vi "zad3.vi"() -> ()   [LabVIEW 2017]
panel:
  in  "Tryb awaryjny":bool
  in  "stop":bool
  out "Lampa Uliczna":cluster{"1":bool, "2":bool, "3":bool}
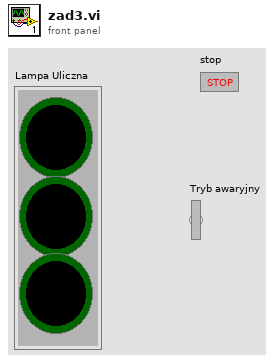
[diagram p1: front panel]
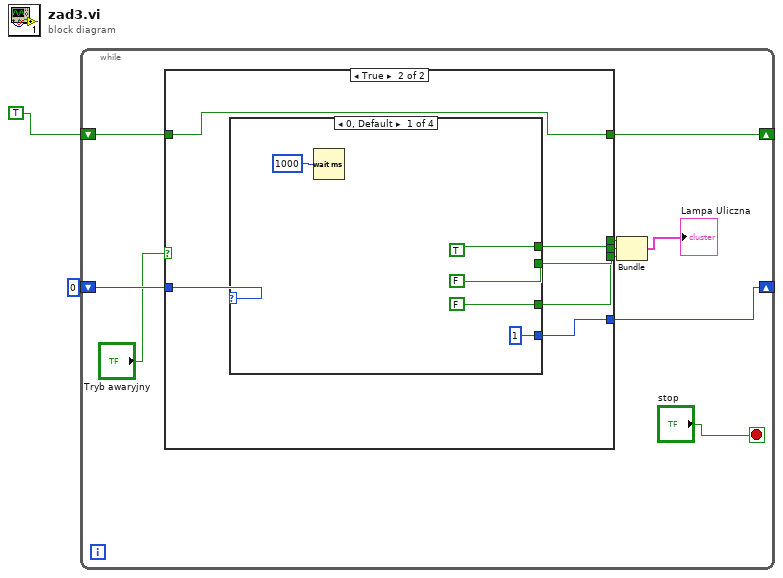
[diagram p0: block diagram]
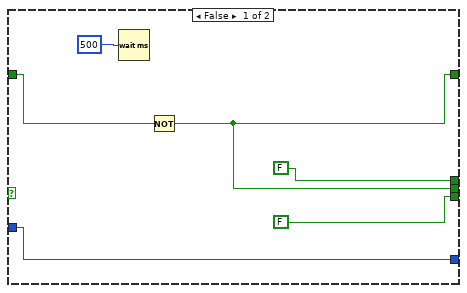
[diagram p2: hidden frame]
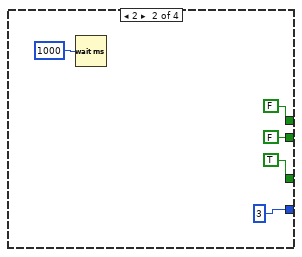
[diagram p3: hidden frame]
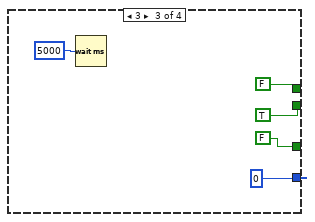
[diagram p4: hidden frame]
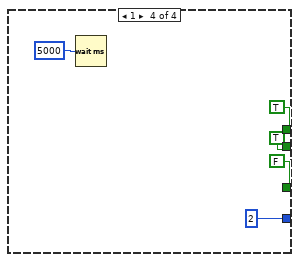
[diagram p5: hidden frame]
diagram:
  n1 = while {
    shift-right: [w6] -> _
    shift-left: 0 -> [w7]
    shift-right: [w3] -> _
    shift-left: TRUE ("2") -> [w4]
    stop <- "stop" stop-if-true
    n2 = case shown="True" "Tryb awaryjny" {
      tunnel: [w13 w24] -> w11
      tunnel: [FALSE ("3") w23] -> w10
      tunnel: [FALSE ("1") w22] -> w9
      tunnel: w7 -> [w16 w21]
      tunnel: [w16 w20] -> w6
      tunnel: [w13 w19] -> w3
      tunnel: w4 -> [w14 w19]
      frame False {
        n3 = Wait (ms)(milliseconds to wait=500) -> ()  [unwired: 1 out]
        n4 = Not(x=w14) -> (.not. x?=w13:bool)
      }
      frame True {
        n5 = case shown="0, Default" w21 {
          tunnel: [FALSE ("2") FALSE ("2") TRUE ("2") TRUE ("2")] -> w24
          tunnel: [FALSE ("3") TRUE ("3") FALSE ("3") FALSE ("3")] -> w23
          tunnel: [TRUE ("1") FALSE ("1") FALSE ("1") TRUE ("1")] -> w22
          tunnel: [1 3 0 2] -> w20
          frame 0, Default {
            n6 = Wait (ms)(milliseconds to wait=1000) -> ()  [unwired: 1 out]
          }
          frame 2 {
            n7 = Wait (ms)(milliseconds to wait=1000) -> ()  [unwired: 1 out]
          }
          frame 3 {
            n8 = Wait (ms)(milliseconds to wait=5000) -> ()  [unwired: 1 out]
          }
          frame 1 {
            n9 = Wait (ms)(milliseconds to wait=5000) -> ()  [unwired: 1 out]
          }
        }
      }
    }
    n10 = Bundle("1"=w9, "2"=w11, "3"=w10) -> (→"Lampa Uliczna":cluster{"1":bool, "2":bool, "3":bool})  [unwired: 1 in]
  }
